vi "AddText.vi"(8 "error in":errorcluster, 9 "Text":string, 10 "OwningElement in":refnum<k20>, 11 "Document in":refnum<k20>) -> (0 "error out":errorcluster, 2 "OwningElement out":refnum<k20>, 3 "Document out":refnum<k20>)   [LabVIEW 2021, in "ProligentXMLGenerator.lvlib" / "DOMSupport.lvlib"]
uses:
  DOMSupport.lvlib
  <resource>/objmgr/DOMUserDefRef.rc
  <vilib>/xml/NI_XML.lvlib
  <vilib>/xml/Close Reference(Node).vi
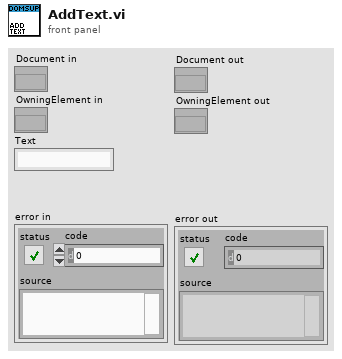
[diagram p1: front panel]
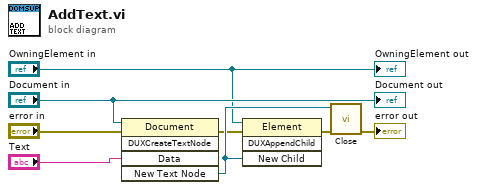
[diagram p0: block diagram]
diagram:
  n1 = invoke on="Invoke Node" class="Document" method="DUXCreateTextNode"(reference="Document in", error in="error in", "Data"="Text") -> (error out=w5:errorcluster, "New Text Node"=w8:refnum<k20>)  [unwired: 2 in, 3 out]
  n2 = invoke on="Invoke Node" class="Element" method="DUXAppendChild"(reference="OwningElement in", error in=w5, "New Child"=w8) -> (error out=w6:errorcluster)  [unwired: 1 in, 3 out]
  n3 = call-poly <vilib>:"Close.vi"("error in (no error)"=w6, "node"=w8) -> ("error out"=→"error out":errorcluster)  [unwired: 7 in]
  "Document out" <- "Document in"
  "OwningElement out" <- "OwningElement in"
